vi "StartHioki.vi"(7 "TimeOut":u32=300, 8 "error in (no error)":errorcluster) -> (0 "ErrSRT":errorcluster, 2 "IRoutput":string, 3 "result":dbl[](array[numeric]))   [LabVIEW 2016]
uses:
  DISGradingMachine/global value.vi
  meter global.vi
  <vilib>/Instr/_visa.llb/VISA Configure Serial Port (Instr).vi
panel:
  out "error out":errorcluster
  out "read buffer":string
  out "Measure time":u32
  out "x-y":u32
  out "ReadErr":bool caption="讀取失敗"
  # "IR量測中,請稍候........"
  # "升壓中,高壓危險 請勿觸碰測座"
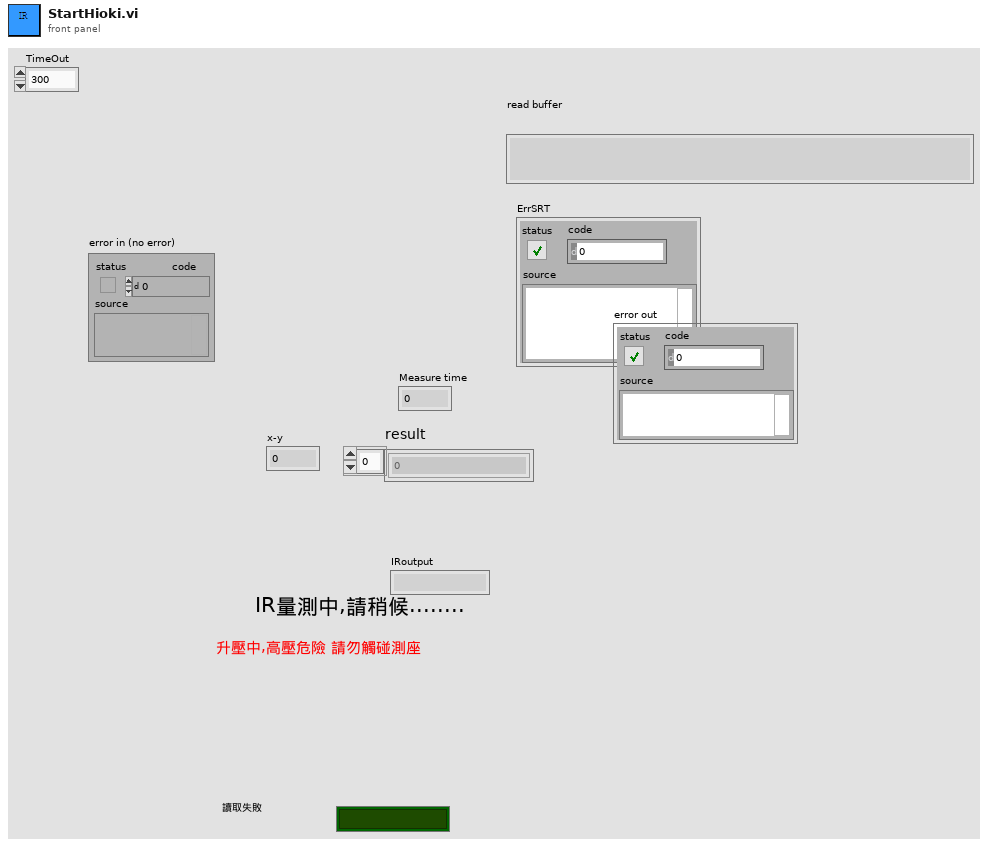
[diagram p1: front panel]
types:
  T1 = enum16{"RDT?", "IDN?", "SRT", "CBF", "SEQ?", "RMT", "SEQ", "PWS", "STP", "PWS?", "PWA", "CHS", ""}
  T2 = enum16{"RDT?", "IDN?", "SRT", "CBF", "SEQ?", "RMT", "SEQ", "PWS", "STP", "PWS?"}
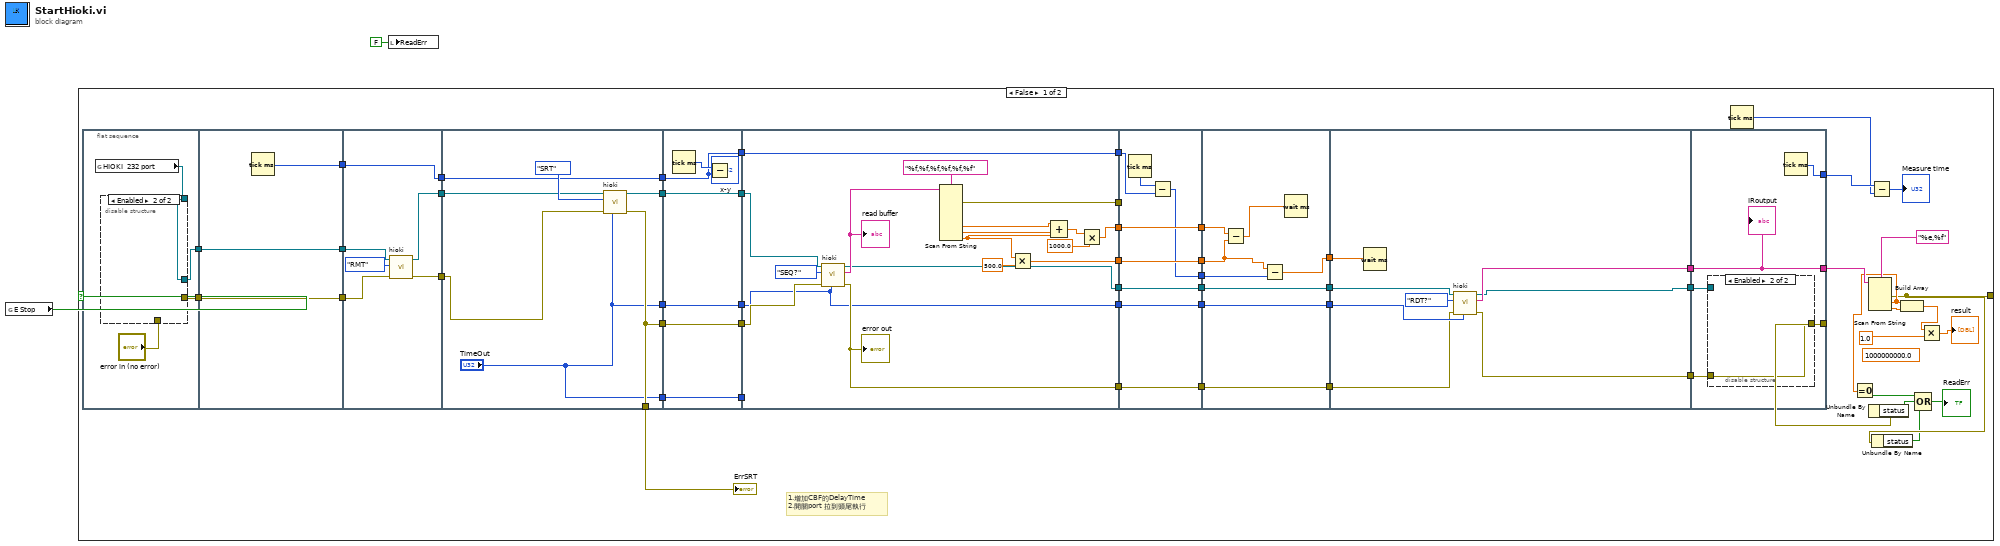
[diagram p0: block diagram]
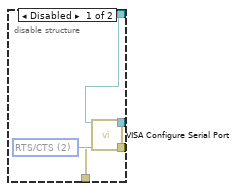
[diagram p2: hidden frame]
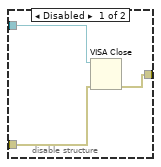
[diagram p3: hidden frame]
diagram:
  n1 = global read "global value.vi" "E Stop"() -> (w2:bool)
  n2 = case shown="False" w2 {
    tunnel: [w19 _] -> _
    frame False {
      (unwired) 1000000000.0
      # "1.增加CBF的DelayTime\n2.開關port 拉到頭尾執行"
      n3 = flat-sequence {
        tunnel: [w61] -> w41
        tunnel: [w60] -> w39
        tunnel: w41 -> [w70]
        tunnel: [w70] -> w40
        tunnel: w39 -> [w69]
        tunnel: [w69] -> w38
        tunnel: [w68] -> w24
        tunnel: [w75] -> w56
        tunnel: w40 -> [w74]
        tunnel: w38 -> [w73]
        tunnel: [w72] -> w55
        tunnel: [w71] -> w43
        tunnel: w24 -> [w71]
        tunnel: ["TimeOut"] -> w54
        tunnel: [w80] -> w57
        tunnel: w56 -> [w79]
        tunnel: w55 -> [w82]
        tunnel: [w81] -> w52
        tunnel: [w80] -> w50
        tunnel: ["TimeOut"] -> w45
        tunnel: w43 -> [w77]
        tunnel: [w77] -> w42
        tunnel: w54 -> [w90]
        tunnel: [w90] -> w53
        tunnel: w52 -> [w89]
        tunnel: [w89] -> w51
        tunnel: w50 -> [w88]
        tunnel: [w88] -> w49
        tunnel: w45 -> [w87]
        tunnel: [w87] -> w44
        tunnel: w42 -> [w84]
        tunnel: [w84] -> w6
        tunnel: w53 -> [w101]
        tunnel: w51 -> [w106]
        tunnel: w49 -> [w105]
        tunnel: [w103] -> w16
        tunnel: [w102] -> w14
        tunnel: w44 -> [_]
        tunnel: [w101] -> w12
        tunnel: [w96] -> w10
        tunnel: [w93] -> w8
        tunnel: w6 -> [w92]
        tunnel: [w92] -> w5
        tunnel: [w91] -> w3
        tunnel: w16 -> [w116]
        tunnel: [w116] -> w15
        tunnel: w14 -> [w115]
        tunnel: [w115] -> w13
        tunnel: w12 -> [w114]
        tunnel: [w114] -> w11
        tunnel: w10 -> [w113]
        tunnel: [w113] -> w9
        tunnel: w8 -> [w112]
        tunnel: [w112] -> w7
        tunnel: w5 -> [w110]
        tunnel: [w109] -> w4
        tunnel: w3 -> [_]
        tunnel: w15 -> [w124]
        tunnel: [w124] -> w37
        tunnel: w13 -> [w123]
        tunnel: [w123] -> w36
        tunnel: [w122] -> w35
        tunnel: w11 -> [w122]
        tunnel: w9 -> [w121]
        tunnel: w7 -> [w119]
        tunnel: [w117] -> w25
        tunnel: w4 -> [w118]
        tunnel: w37 -> [w131]
        tunnel: [w126] -> w48
        tunnel: w36 -> [w128]
        tunnel: [w129] -> w47
        tunnel: [w127] -> w46
        tunnel: w35 -> [w130]
        tunnel: w25 -> [w125]
        tunnel: [w137] -> w34
        tunnel: w48 -> [w136]
        tunnel: w47 -> [w137]
        tunnel: w46 -> [w135]
        tunnel: [w134] -> w28
        tunnel: [w133] -> w21
        frame #0 {
          n4 = global read "meter global.vi" "HIOKI  232 port"() -> (w59:refnum<visa-resource-name>)
          n5 = disable-structure shown="Enabled" {
            disable-tunnel: [w66 w67] -> w61
            disable-tunnel: [w65 _] -> w60
            disable-tunnel: w59 -> [w64 w67]
            disable-tunnel: "error in (no error)" -> [w62 _]
            frame Disabled {
              w63 = u16 2 items=["None", "XON/XOFF", "RTS/CTS", "XON/XOFF & RTS/CTS", "DTR/DSR", "XON/XOFF & DTR/DSR"] ("flow control (0:none)")
              n6 = call-poly "VISA Configure Serial Port"("VISA resource name"=w64, "error in (no error)"=w62, "flow control (0:none)"=w63) -> ("VISA resource name out"=w66:refnum<visa-resource-name>, "error out"=w65:errorcluster)  [unwired: 11 in]
            }
            frame Enabled {
            }
          }
        }
        frame #1 {
          n7 = Tick Count (ms)() -> (millisecond timer value=w68:u32)
        }
        frame #2 {
          n8 = call "hioki.vi"("error in (no error)"=w73, "EnumFunction"=T1."RMT", "VISA resource name out"=w74) -> ("error out"=w75:errorcluster, "Visa_HiokiMeterOut"=w72:refnum<visa-resource-name>)  [unwired: 6 in, 1 out]
        }
        frame #3 {
          n9 = call "hioki.vi"("TimeOut"="TimeOut", "error in (no error)"=w79, "EnumFunction"=T2."SRT", "VISA resource name out"=w82) -> ("error out"=w80:errorcluster, "Visa_HiokiMeterOut"=w81:refnum<visa-resource-name>)  [unwired: 5 in, 1 out]
        }
        frame #4 {
          n10 = Tick Count (ms)() -> (millisecond timer value=w86:u32)
          n11 = Subtract(x=w86, y=w84) -> (x-y=→"x-y":u32)
        }
        frame #5 {
          n12 = call "hioki.vi"("TimeOut"=w101, "error in (no error)"=w105, "EnumFunction"=T1."SEQ?", "VISA resource name out"=w106) -> ("error out"=w102:errorcluster, "read buffer"=w104:string, "Visa_HiokiMeterOut"=w103:refnum<visa-resource-name>)  [unwired: 5 in]
          "read buffer" <- w104
          "error out" <- w102
          n13 = Scan From String(format string="%f,%f,%f,%f,%f,%f", input string=w104) -> (error out=w91:errorcluster, output 4=w100:dbl, output 5=w99:dbl, output 6=w95:dbl)  [unwired: 11 in, 2 out]
          n14 = Multiply(x=w95, y=500.0) -> (x*y=w93:dbl)
          n15 = Compound Arithmetic op=ADD(w100, w99, w95) -> (w98:dbl)
          n16 = Multiply(x=w98, y=1000.0) -> (x*y=w96:dbl)
        }
        frame #6 {
          n17 = Tick Count (ms)() -> (millisecond timer value=w111:u32)
          n18 = Subtract(x=w111, y=w110) -> (x-y=w109:u32)
        }
        frame #7 {
          n19 = Subtract(x=w121, y=w119) -> (x-y=w120:dbl)
          n20 = Subtract(x=w119, y=w118) -> (x-y=w117:dbl)
          n21 = Wait (ms)(milliseconds to wait=w120) -> ()  [unwired: 1 out]
        }
        frame #8 {
          n22 = Wait (ms)(milliseconds to wait=w125) -> ()  [unwired: 1 out]
          n23 = call "hioki.vi"("TimeOut"=w130, "error in (no error)"=w128, "EnumFunction"=T1."RDT?", "VISA resource name out"=w131) -> ("error out"=w127:errorcluster, "read buffer"=w129:string, "Visa_HiokiMeterOut"=w126:refnum<visa-resource-name>)  [unwired: 5 in]
        }
        frame #9 {
          n24 = disable-structure shown="Enabled" {
            disable-tunnel: w136 -> [w140 _]
            disable-tunnel: w135 -> [w139 w141]
            disable-tunnel: [w138 w141] -> w133
            frame Disabled {
              n25 = VISA Close(VISA resource name=w140, error in (no error)=w139) -> (error out=w138:errorcluster)
            }
            frame Enabled {
            }
          }
          n26 = Tick Count (ms)() -> (millisecond timer value=w134:u32)
          "IRoutput" <- w137
        }
      }
      n27 = Tick Count (ms)() -> (millisecond timer value=w27:u32)
      n28 = Unbundle By Name(w21) -> ("status"=w20:bool)
      n29 = Scan From String(format string="%e,%f", input string=w34) -> (error out=w19:errorcluster, output 1=w22:dbl, output 2=w32:dbl)  [unwired: 4 in, 2 out]
      n30 = Equal To 0?(x=w22) -> (x = 0?=w23:bool)
      n31 = Subtract(x=w28, y=w27) -> (x-y=→"Measure time":u32)
      n32 = Unbundle By Name(w19) -> ("status"=w18:bool)
      n33 = Build Array(w22, w32) -> (w31:dbl[])
      n34 = Compound Arithmetic op=OR(w23, w20, w18) -> (→"ReadErr":bool)
      n35 = Multiply(x=w31, y=1.0) -> (x*y=→"result":dbl[])
      "ErrSRT" <- w57
    }
    frame True {
    }
  }
  n36 = local write "ReadErr"(FALSE ("ReadErr")) -> ()
